vi "main.vi"(8 "error in (no error)":errorcluster) -> (0 "error out":errorcluster)   [LabVIEW 2015, in "Sample.lvlib"]
doc: "使用该模板构建用户界面事件处理设计模式。将模板应用于对话框及其它用户界面。用户也可创建并执行VI可按照与用户界面事件相同方式处理的用户定义事件。"
uses:
  Sample.lvlib
  Support/Result Panel State.ctl
  Support/UI Ref.ctl
  <vilib>/addons/database/Connection.llb/Conn ObjectReference.ctl
  Support/Configuration.ctl
  Sub VIs/Database Processing/Support/Table/Measure_Bio_Type.ctl
  Sub VIs/Database Processing/Database Processing.lvlib
  <vilib>/addons/database/NI_Database_API.lvlib
  Sub VIs/Utility VIs/Utility VIs.lvlib
  Sub VIs/Boimetry Processing/Boimetry Processing.lvlib
panel:
  in  "计算":bool caption="开始"
  in  "开始":bool
  in  "编辑":bool caption="开始"
  out "出生日期":string
  out "性别":string
  out "姓名":string
  in  "OD Summary":string[][](table)
  in  "OD parameter list":string[][](table)
  out "Image":T1(plugin-control)
  out "Ascan Display":dbl[](graph)
  in  "OS Summary":string[][](table)
  in  "OS parameter list":string[][](table)
  out "状态栏":string
  in  "stop":bool caption="停止"
  # "WJ90000生物参数测量仪"
  # "OD"
  # "OS"
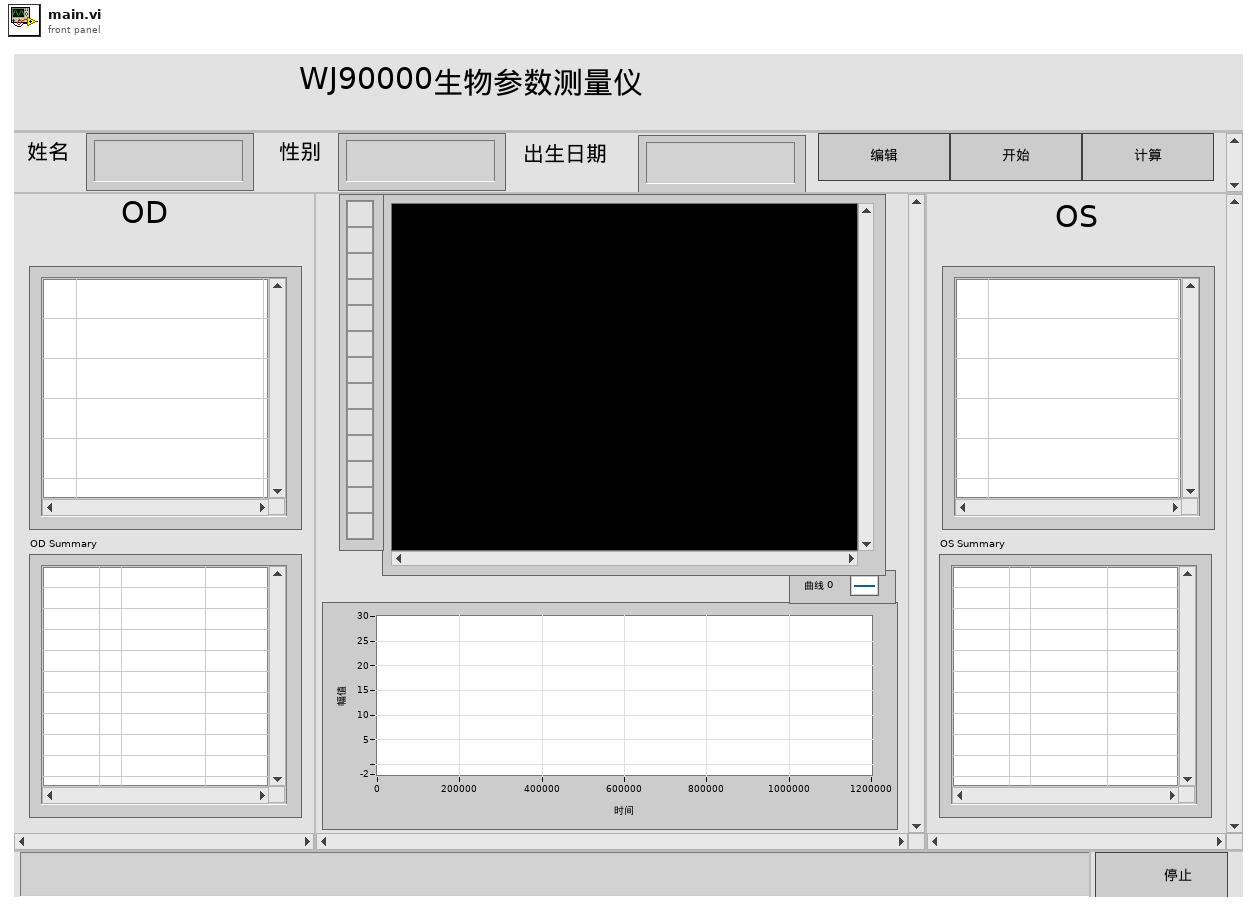
[diagram p1: front panel]
types:
  T1 = typedef "IMAQ Image.ctl" = refnum<image>
  T2 = typedef "Sample.lvlib/Configuration.ctl" = cluster{"Measure_No":i64, "Patient_ID":i64, "Oridinal":i64, "Display Parameter":enum16{"CCT", "ACD", "LT", "RT", "AL", "PD", "WTW", "K_flat", "K_steep", "K_AST"}}
  T3 = typedef "NI_Database_API.lvlib/Conn ObjectReference.ctl" = refnum<k1>
  T4 = typedef "Sample.lvlib/UI Ref.ctl" = cluster{"编辑引用句柄":refnum<vi>, "开始引用句柄":refnum<vi>, "停止引用句柄":refnum<vi>, "Ascan引用句柄":refnum<vi>, "OD Summary引用句柄":refnum<vi>, "OS Summary引用句柄":refnum<vi>, "OD parameter list引用句柄":refnum<vi>, "OS parameter list引用句柄":refnum<vi>}
  T5 = typedef "Sample.lvlib/Result Panel State.ctl" = enum16{"Initialize", "Connect Database", "Select Database", "Register", "Wait For Event", "Start", "Calculation", "Display Result", "OS Summary Update", "OS Parameter List Update", "OD Summary Update", "OD Parameter List Update", "Exit", "OD IMG Parameter List Update", "OS IMG Parameter List Update"}
  T6 = typedef "Database Processing.lvlib/Measure_Bio_Type.ctl" = cluster{"Measure_No":i64, "Measure_Time":string, "Patient_ID":i64}
  T7 = enum16{"CCT", "ACD", "LT", "RT", "AL", "PD", "WTW", "K_flat", "K_steep", "K_AST"}
  T8 = typedef "LVPoint32TypeDef.ctl" = cluster{"Horizontal":i32, "Vertical":i32}
  T9 = typedef "LVRowAndColumnTypeDef.ctl" = cluster{"Row":i32, "Column":i32}
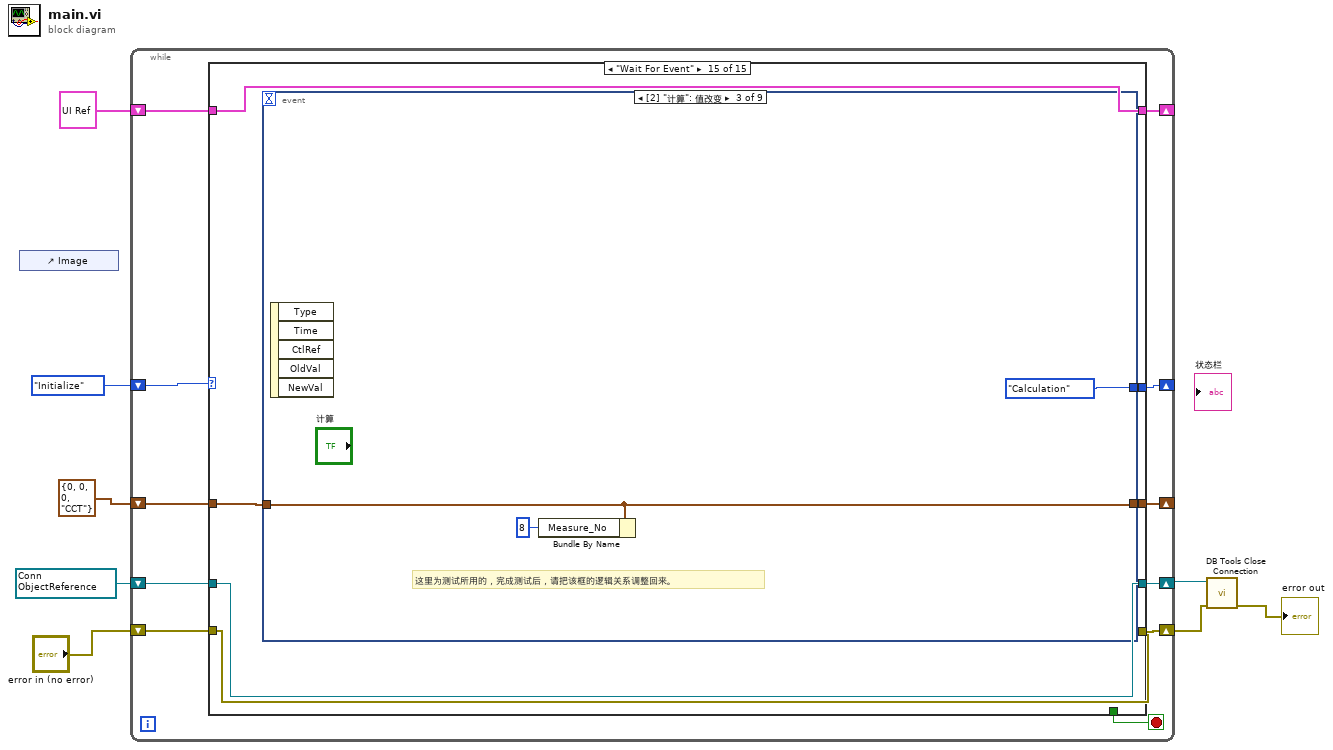
[diagram p0: block diagram]
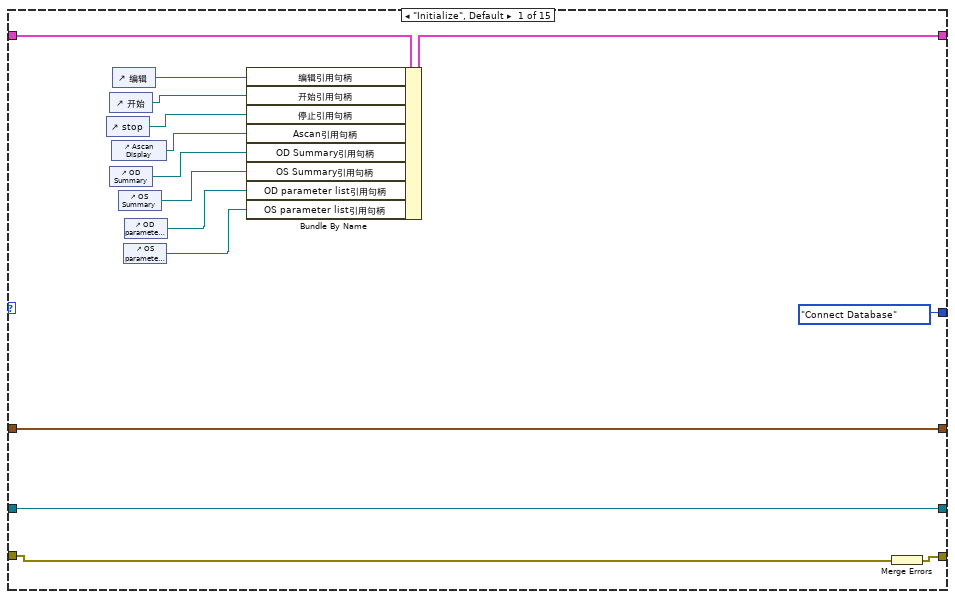
[diagram p2: hidden frame]
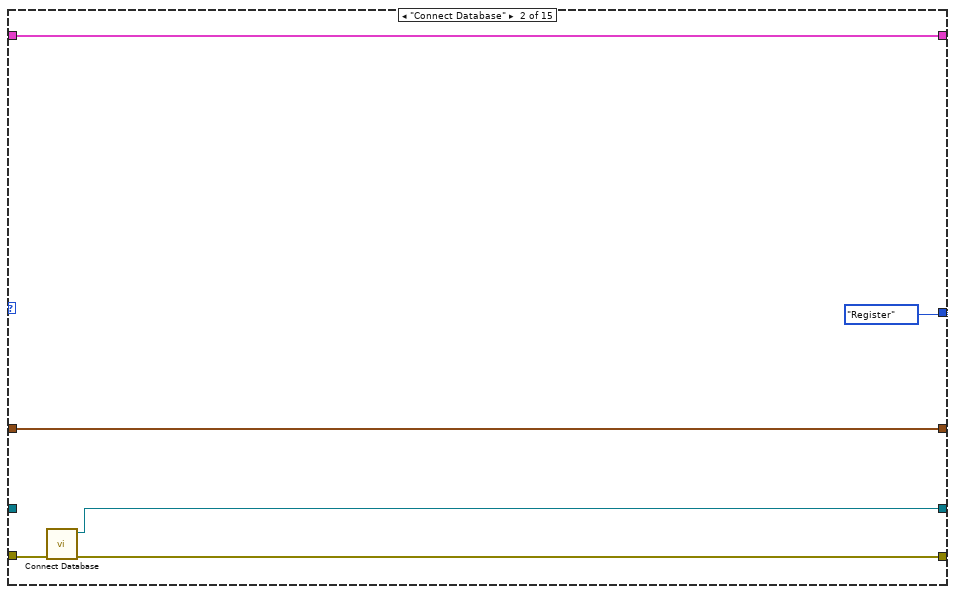
[diagram p3: hidden frame]
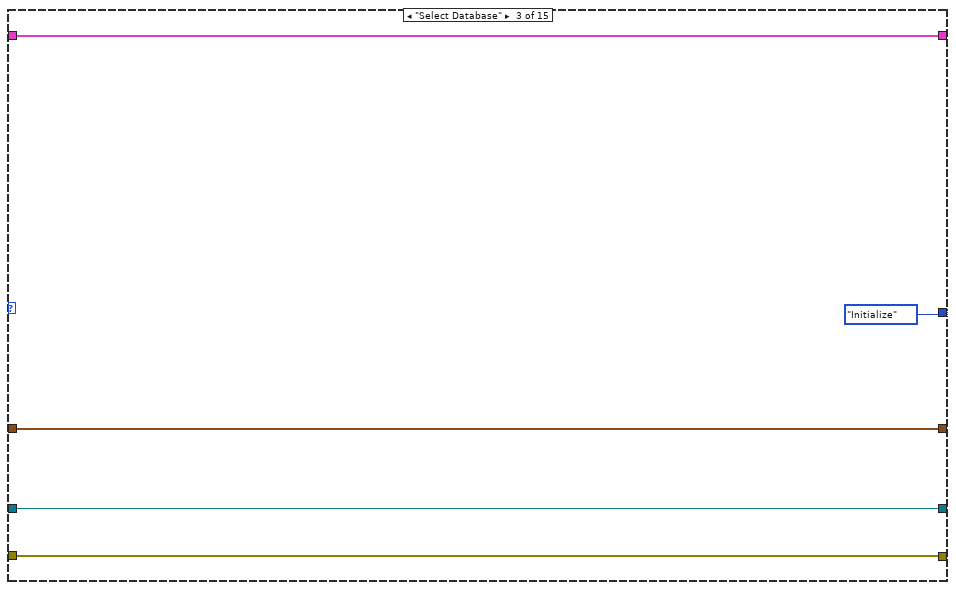
[diagram p4: hidden frame]
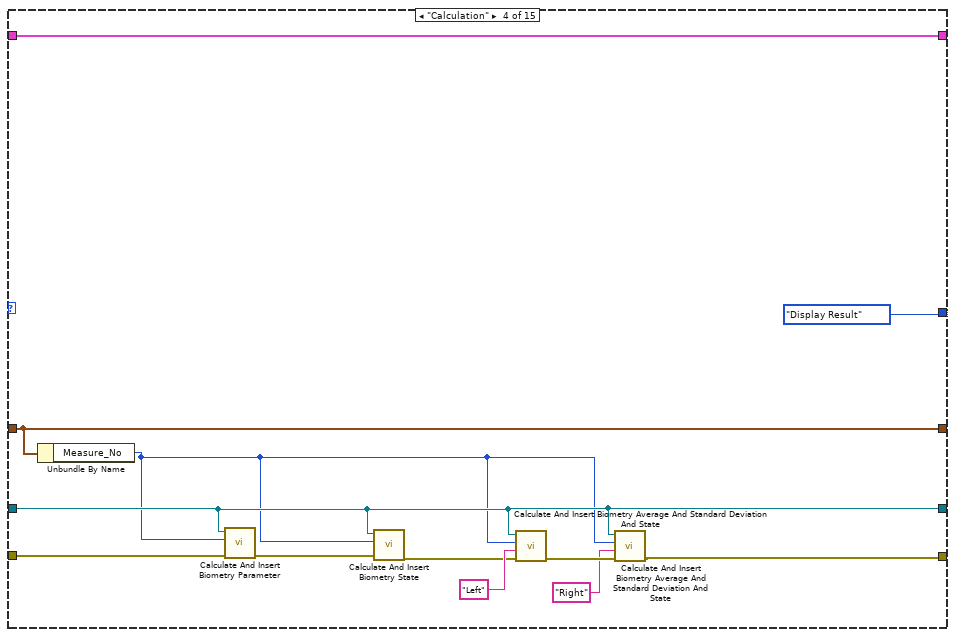
[diagram p5: hidden frame]
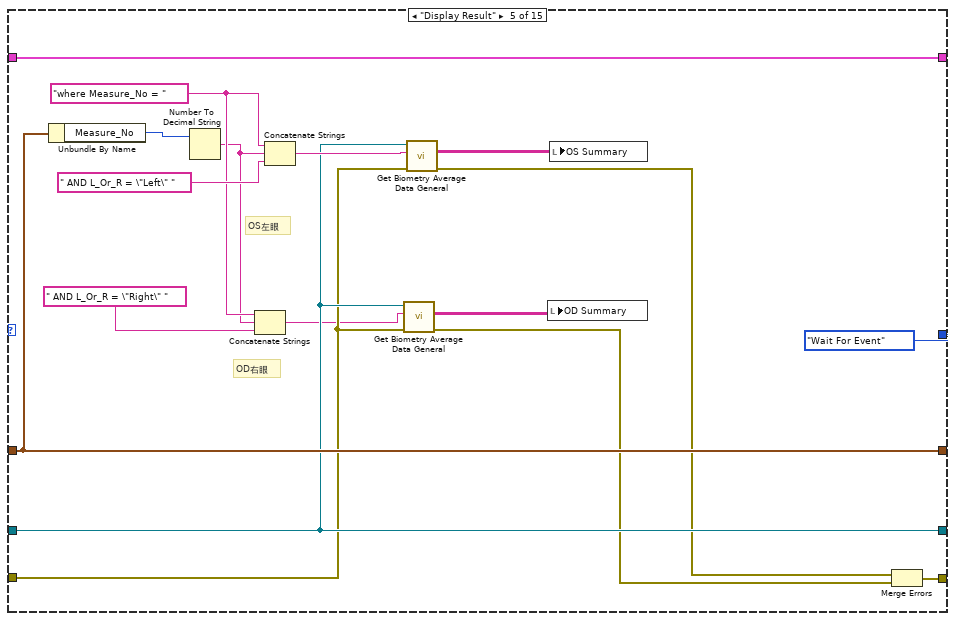
[diagram p6: hidden frame]
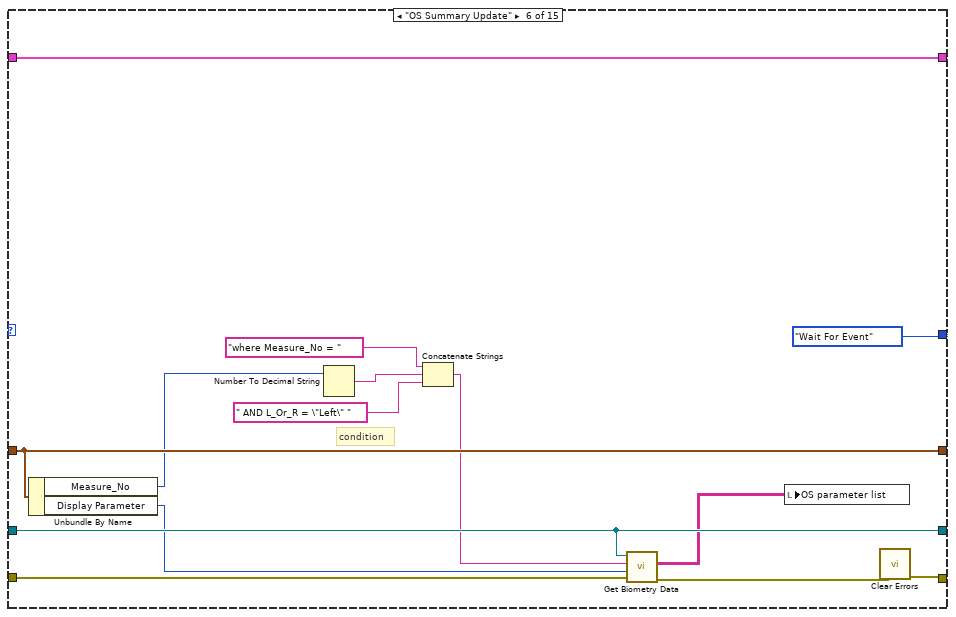
[diagram p7: hidden frame]
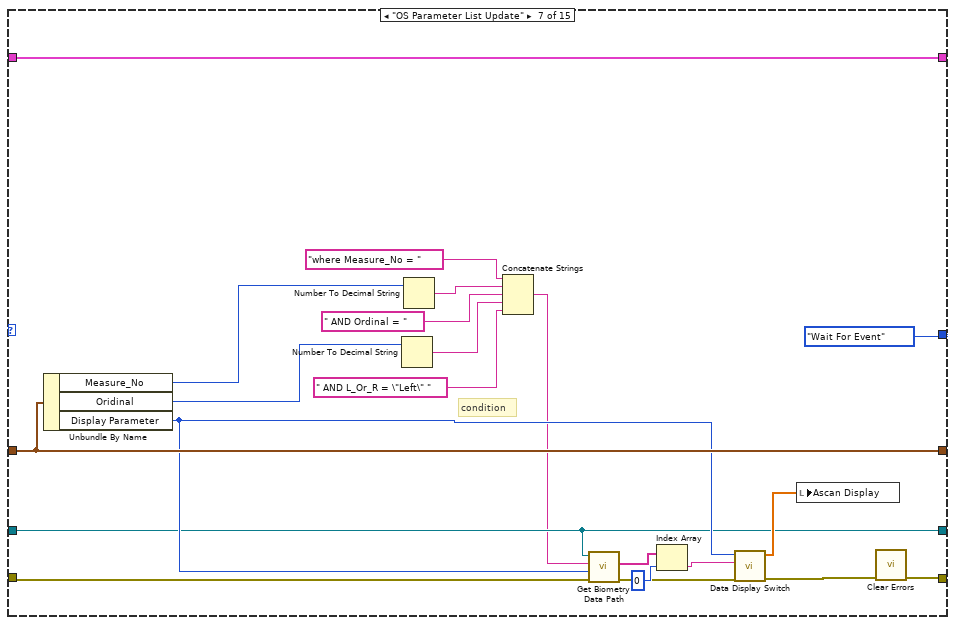
[diagram p8: hidden frame]
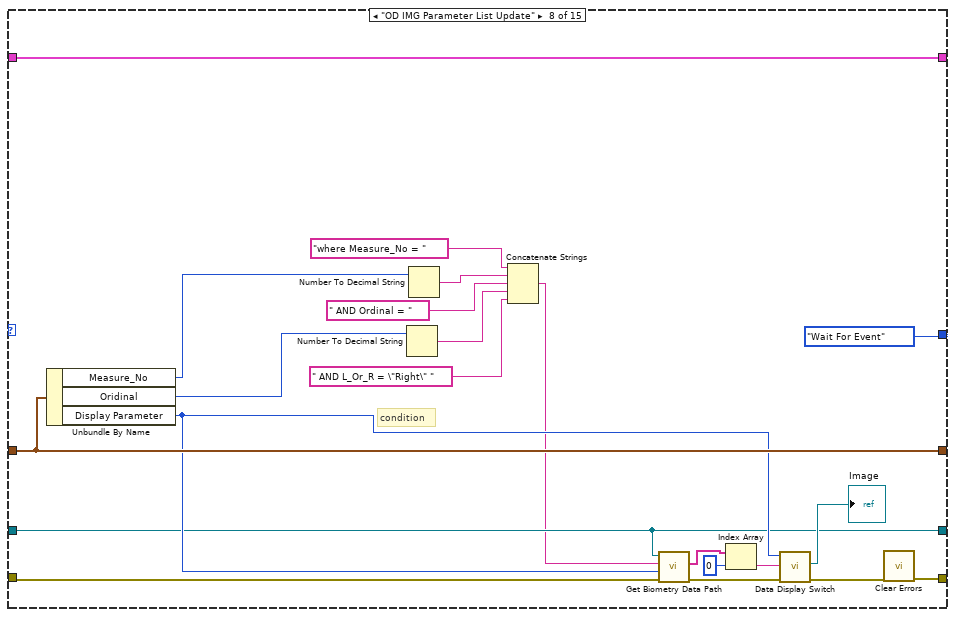
[diagram p9: hidden frame]
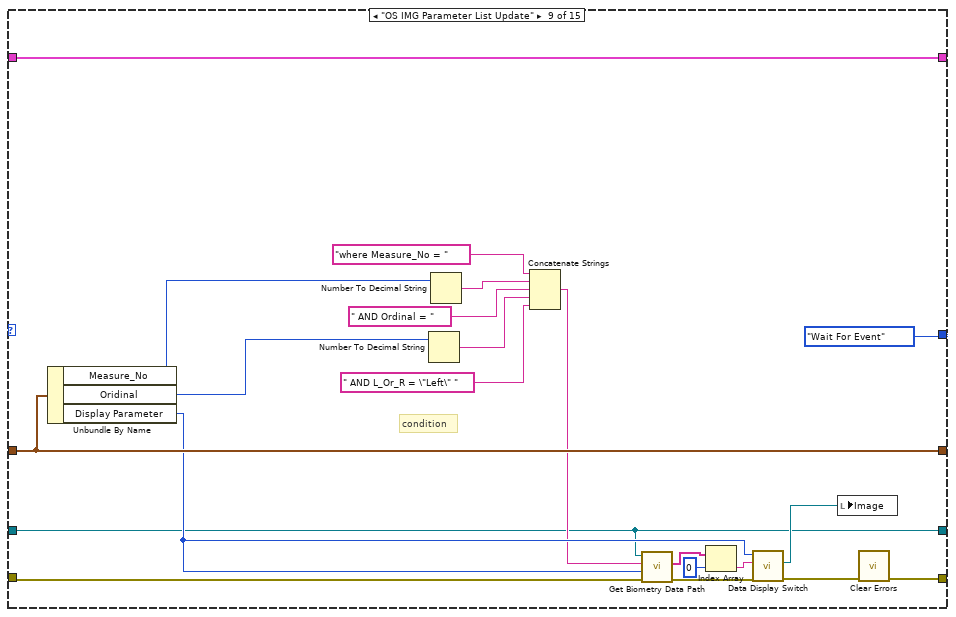
[diagram p10: hidden frame]
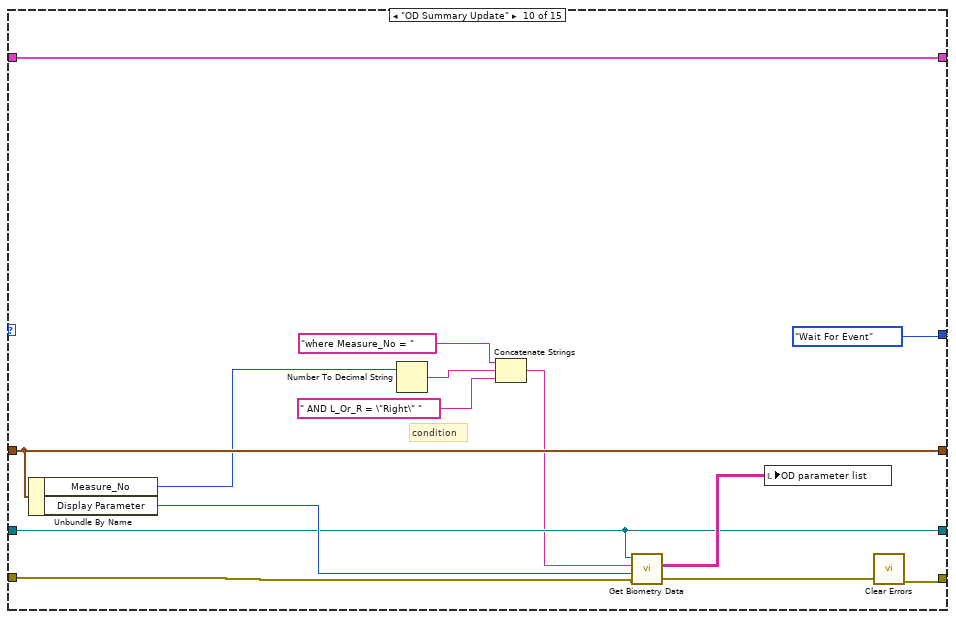
[diagram p11: hidden frame]
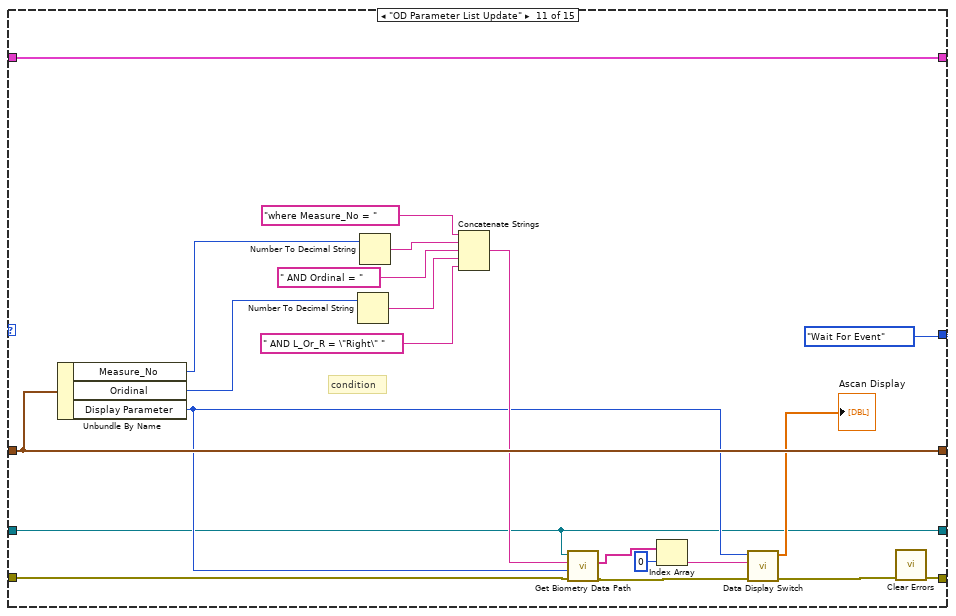
[diagram p12: hidden frame]
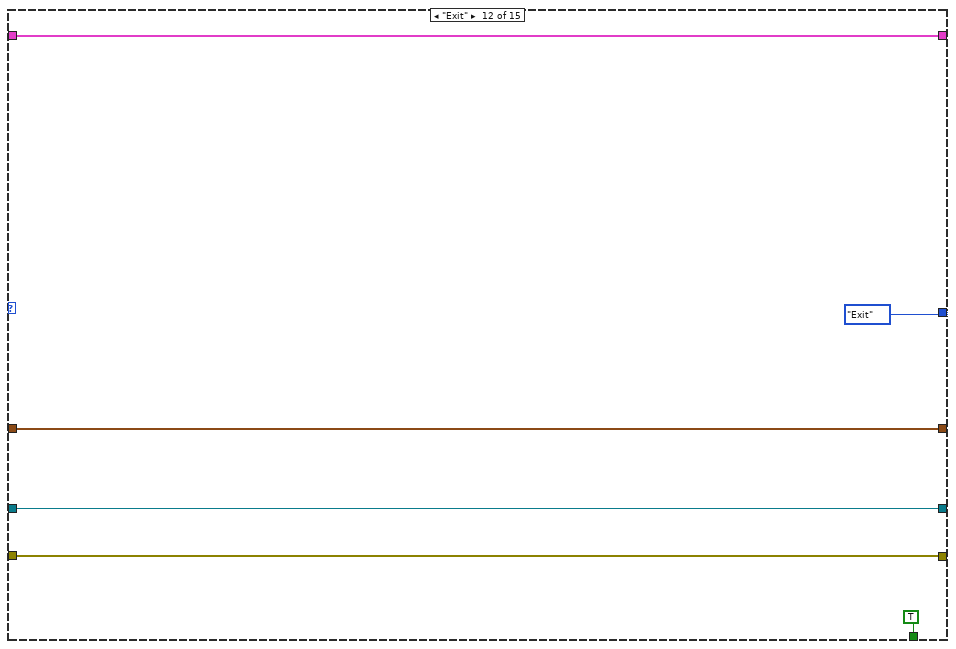
[diagram p13: hidden frame]
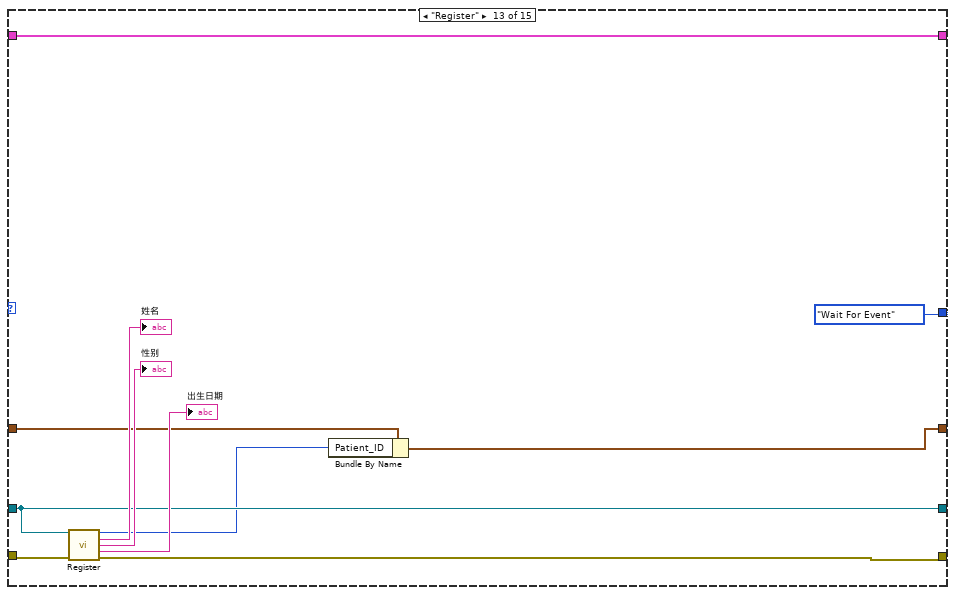
[diagram p14: hidden frame]
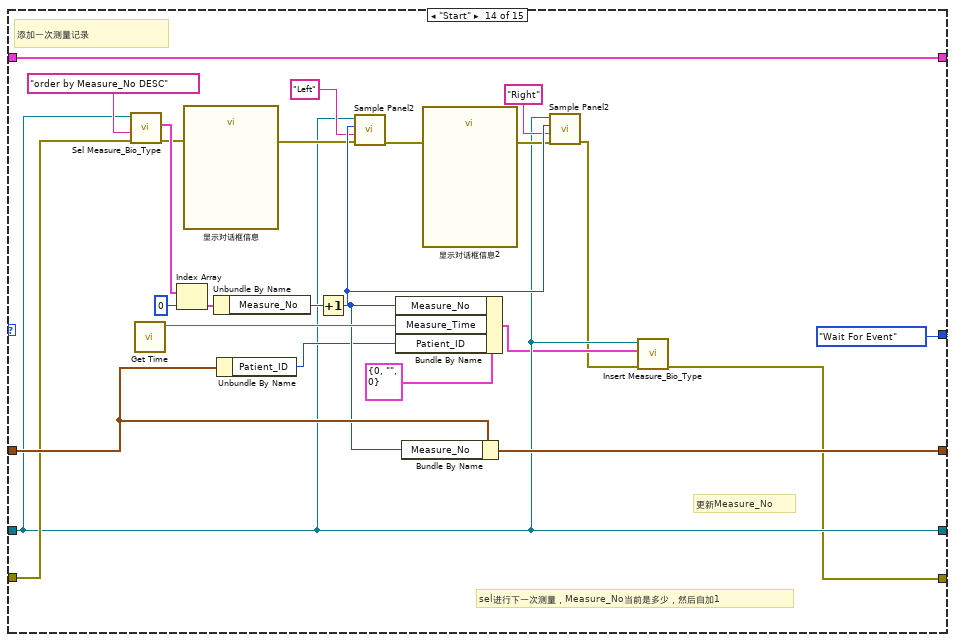
[diagram p15: hidden frame]
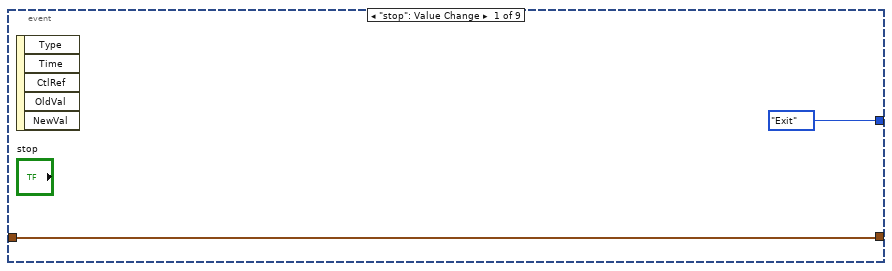
[diagram p16: hidden frame]
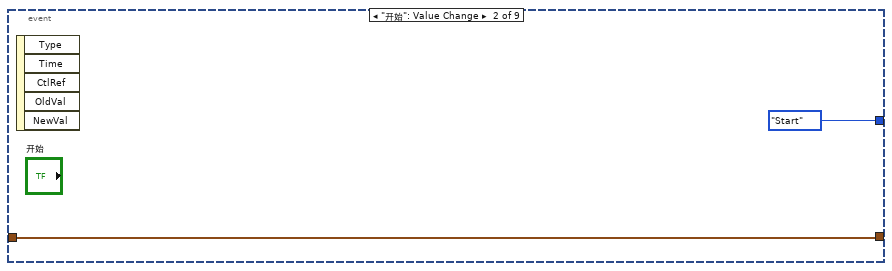
[diagram p17: hidden frame]
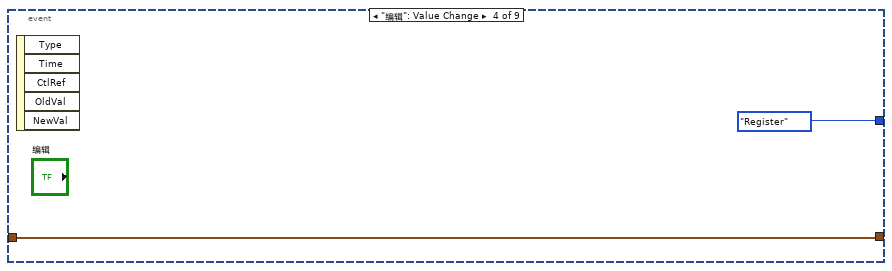
[diagram p18: hidden frame]
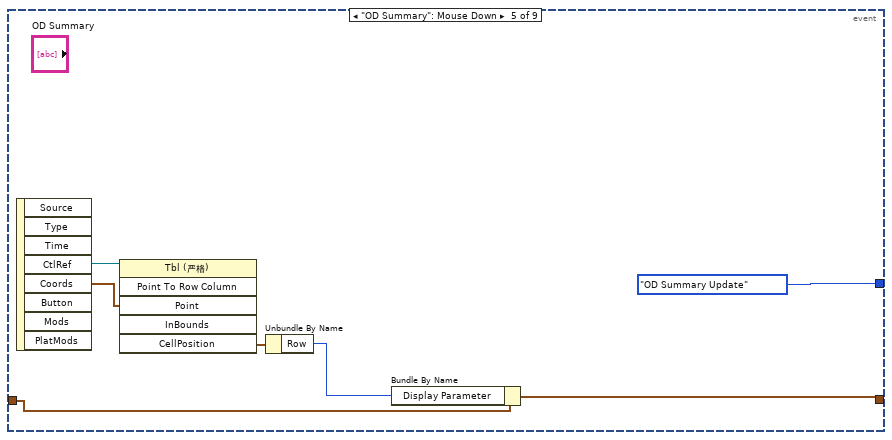
[diagram p19: hidden frame]
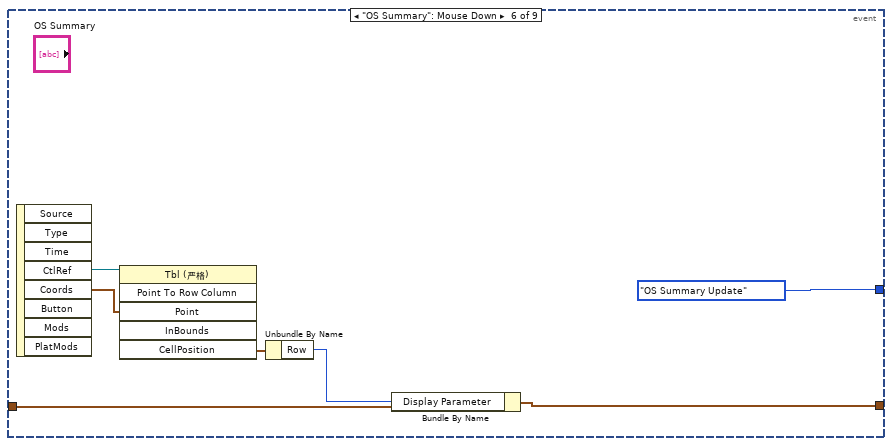
[diagram p20: hidden frame]
diagram:
  w5 = T3 refnum items=["Connection"] ("connection reference")
  n1 = control-ref of="Image"() -> ()  [unwired: 1 out]
  n2 = while {
    shift-right: [w17] -> _
    shift-left: T4 {"编辑引用句柄"=refnum, "开始引用句柄"=refnum, "停止引用句柄"=refnum, "Ascan引用句柄"=refnum, "OD Summary引用句柄"=refnum, "OS Summary引用句柄"=refnum, "OD parameter list引用句柄"=refnum, "OS parameter list引用句柄"=refnum} ("UI State") -> [w16]
    shift-right: [w15] -> _
    shift-left: Result_Panel_State."Initialize" ("State") -> [w18]
    shift-right: [w13] -> w3
    shift-left: "error in (no error)" -> [w14]
    shift-right: [w11] -> _
    shift-left: T2 {"Measure_No"=0, "Patient_ID"=0, "Oridinal"=0, "Display Parameter"=enum."CCT"} ("Configuration") -> [w12]
    shift-right: [w9] -> w4
    shift-left: w5 -> [w10]
    stop <- w19 stop-if-true
    n3 = case shown="\"Wait For Event\"" w18 {
      tunnel: [_ _ _ _ _ _ _ _ _ _ _ TRUE ("stop") _ _ _] -> w19
      tunnel: [w29 w37 w45 w57 w66 w85 w109 w130 w151 w162 w186 w192 w201 w226 w230] -> w17
      tunnel: w16 -> [w34 w37 w45 w57 w66 w85 w109 w130 w151 w162 w186 w192 w201 w226 w230]
      tunnel: [Result_Panel_State."Connect Database" ("State") Result_Panel_State."Register" ("State") Result_Panel_State."Initialize" ("State") Result_Panel_State."Display Result" ("State") Result_Panel_State."Wait For Event" ("State") Result_Panel_State."Wait For Event" ("State") Result_Panel_State."Wait For Event" ("State") Result_Panel_State."Wait For Event" ("State") Result_Panel_State."Wait For Event" ("State") Result_Panel_State."Wait For Event" ("State") Result_Panel_State."Wait For Event" ("State") Result_Panel_State."Exit" ("State") Result_Panel_State."Wait For Event" ("State") Result_Panel_State."Wait For Event" ("State") w233] -> w15
      tunnel: w14 -> [w20 w39 w41 w55 w63 w84 w101 w119 w140 w160 w172 w188 w202 w211 w232]
      tunnel: [w21 w38 w41 w49 w73 w86 w103 w124 w145 w163 w180 w188 w196 w204 w232] -> w13
      tunnel: w12 -> [w27 w35 w43 w54 w68 w87 w107 w128 w149 w164 w184 w190 w195 w224 w229]
      tunnel: [w27 w35 w43 w54 w68 w87 w107 w128 w149 w164 w184 w190 w193 w225 w228] -> w11
      tunnel: w10 -> [w26 _ w42 w48 w64 w82 w99 w118 w131 w157 w168 w189 w197 w207 w231]
      tunnel: [w26 w36 w42 w48 w64 w82 w99 w118 w131 w157 w168 w189 w197 w207 w231] -> w9
      frame "Initialize", Default {
        n4 = control-ref of="stop"() -> (w31:refnum<vi>)
        n5 = control-ref of="开始"() -> (w32:refnum<vi>)
        n6 = control-ref of="OD Summary"() -> (w25:refnum<vi>)
        n7 = control-ref of="Ascan Display"() -> (w30:refnum<vi>)
        n8 = control-ref of="编辑"() -> (w33:refnum<vi>)
        n9 = control-ref of="OS Summary"() -> (w24:refnum<vi>)
        n10 = control-ref of="OS parameter list"() -> (w22:refnum<vi>)
        n11 = control-ref of="OD parameter list"() -> (w23:refnum<vi>)
        n12 = Bundle By Name(cluster=w34, "编辑引用句柄"=w33, "开始引用句柄"=w32, "停止引用句柄"=w31, "Ascan引用句柄"=w30, "OD Summary引用句柄"=w25, "OS Summary引用句柄"=w24, "OD parameter list引用句柄"=w23, "OS parameter list引用句柄"=w22) -> (w29:T4)
        n13 = Merge Errors(w20) -> (w21:errorcluster)
      }
      frame "Connect Database" {
        n14 = call "Connect Database.vi"("error in (no error)"=w39) -> ("error out"=w38:errorcluster, "connection reference"=w36:T3)  [unwired: 9 in]
      }
      frame "Select Database" {
      }
      frame "Calculation" {
        n15 = Unbundle By Name(w54) -> ("Measure_No"=w47:i64)
        n16 = call "Calculate And Insert Biometry Parameter.vi"("error in (no error)"=w55, "Measure_No"=w47, "connection reference"=w48) -> ("error out"=w53:errorcluster)  [unwired: 8 in]
        n17 = call "Calculate And Insert Biometry State.vi"("error in (no error)"=w53, "Measure_No"=w47, "connection reference"=w48) -> ("error out"=w51:errorcluster)  [unwired: 8 in]
        n18 = call "Calculate And Insert Biometry Average And Standard Deviation And State.vi"("error in (no error)"=w51, "L_Or_R"="Left", "Measure_No"=w47, "connection reference"=w48) -> ("error out"=w50:errorcluster)  [unwired: 7 in]
        n19 = call "Calculate And Insert Biometry Average And Standard Deviation And State.vi"("error in (no error)"=w50, "L_Or_R"="Right", "Measure_No"=w47, "connection reference"=w48) -> ("error out"=w49:errorcluster)  [unwired: 7 in]
      }
      frame "Display Result" {
        w71 = "where Measure_No = " ("字符串")
        # "OD右眼"
        # "OS左眼"
        n20 = Unbundle By Name(w68) -> ("Measure_No"=w67:i64)
        n21 = Number To Decimal String(number=w67) -> (decimal integer string=w70:string)  [unwired: 1 in]
        n22 = Concatenate Strings(w71, w70, " AND L_Or_R = \"Right\" " ("字符串")) -> (w62:string)
        n23 = Concatenate Strings(w71, w70, " AND L_Or_R = \"Left\" " ("字符串")) -> (w65:string)
        n24 = call "Get Biometry Average Data General.vi"("error in (no error)"=w63, "condition"=w62, "connection reference"=w64) -> ("error out"=w58:errorcluster, "Data Output"=w60:string[][])  [unwired: 7 in]
        n25 = call "Get Biometry Average Data General.vi"("error in (no error)"=w63, "condition"=w65, "connection reference"=w64) -> ("error out"=w59:errorcluster, "Data Output"=w61:string[][])  [unwired: 7 in]
        n26 = local write "OD Summary"(w60) -> ()
        n27 = local write "OS Summary"(w61) -> ()
        n28 = Merge Errors(w59, w58) -> (w73:errorcluster)
      }
      frame "OS Summary Update" {
        # "condition"
        n29 = Unbundle By Name(w87) -> ("Measure_No"=w76:i64, "Display Parameter"=w81:T7)
        n30 = Number To Decimal String(number=w76) -> (decimal integer string=w78:string)  [unwired: 1 in]
        n31 = Concatenate Strings("where Measure_No = ", w78, " AND L_Or_R = \"Left\" " ("字符串")) -> (w75:string)
        n32 = call "Get Biometry Data.vi"("error in (no error)"=w84, "Display Parameter"=w81, "condition"=w75, "connection reference"=w82) -> ("error out"=w83:errorcluster, "Data Output"=w80:string[][])  [unwired: 6 in]
        n33 = local write "OS parameter list"(w80) -> ()
        n34 = call <vilib>:"Clear Errors.vi"("error in (no error)"=w83) -> ("error out"=w86:errorcluster)  [unwired: 5 in, 1 out]
      }
      frame "OS Parameter List Update" {
        # "condition"
        n35 = Unbundle By Name(w107) -> ("Measure_No"=w90:i64, "Oridinal"=w89:i64, "Display Parameter"=w100:T7)
        n36 = Number To Decimal String(number=w89) -> (decimal integer string=w95:string)  [unwired: 1 in]
        n37 = Number To Decimal String(number=w90) -> (decimal integer string=w97:string)  [unwired: 1 in]
        n38 = Concatenate Strings("where Measure_No = ", w97, " AND Ordinal = " ("字符串"), w95, " AND L_Or_R = \"Left\" " ("字符串")) -> (w91:string)
        n39 = call "Get Biometry Data Path.vi"("error in (no error)"=w101, "Display Parameter"=w100, "condition"=w91, "connection reference"=w99) -> ("error out"=w102:errorcluster, "Data Path Output"=w93:string[])  [unwired: 6 in]
        n40 = Index Array(array=w93, index=0 ("索引")) -> (element=w92:string)
        n41 = call "Data Display Switch.vi"("error in"=w102, "Path"=w92, "Switch"=w100) -> ("error out"=w104:errorcluster, "Ascan"=w105:dbl[])  [unwired: 6 in, 1 out]
        n42 = local write "Ascan Display"(w105) -> ()
        n43 = call <vilib>:"Clear Errors.vi"("error in (no error)"=w104) -> ("error out"=w103:errorcluster)  [unwired: 5 in, 1 out]
      }
      frame "OD IMG Parameter List Update" {
        # "condition"
        n44 = Unbundle By Name(w128) -> ("Measure_No"=w112:i64, "Oridinal"=w111:i64, "Display Parameter"=w120:T7)
        n45 = Number To Decimal String(number=w111) -> (decimal integer string=w114:string)  [unwired: 1 in]
        n46 = Number To Decimal String(number=w112) -> (decimal integer string=w116:string)  [unwired: 1 in]
        n47 = Concatenate Strings("where Measure_No = ", w116, " AND Ordinal = " ("字符串"), w114, " AND L_Or_R = \"Right\" " ("字符串")) -> (w110:string)
        n48 = call "Get Biometry Data Path.vi"("error in (no error)"=w119, "Display Parameter"=w120, "condition"=w110, "connection reference"=w118) -> ("error out"=w123:errorcluster, "Data Path Output"=w122:string[])  [unwired: 6 in]
        n49 = Index Array(array=w122, index=0 ("索引")) -> (element=w121:string)
        n50 = call "Data Display Switch.vi"("error in"=w123, "Path"=w121, "Switch"=w120) -> ("error out"=w125:errorcluster, "Image Out"=→"Image":T1)  [unwired: 6 in, 1 out]
        n51 = call <vilib>:"Clear Errors.vi"("error in (no error)"=w125) -> ("error out"=w124:errorcluster)  [unwired: 5 in, 1 out]
      }
      frame "OS IMG Parameter List Update" {
        # "condition"
        n52 = Unbundle By Name(w149) -> ("Measure_No"=w133:i64, "Oridinal"=w132:i64, "Display Parameter"=w141:T7)
        n53 = Number To Decimal String(number=w132) -> (decimal integer string=w136:string)  [unwired: 1 in]
        n54 = Number To Decimal String(number=w133) -> (decimal integer string=w138:string)  [unwired: 1 in]
        n55 = Concatenate Strings("where Measure_No = ", w138, " AND Ordinal = " ("字符串"), w136, " AND L_Or_R = \"Left\" " ("字符串")) -> (w134:string)
        n56 = call "Get Biometry Data Path.vi"("error in (no error)"=w140, "Display Parameter"=w141, "condition"=w134, "connection reference"=w131) -> ("error out"=w144:errorcluster, "Data Path Output"=w143:string[])  [unwired: 6 in]
        n57 = Index Array(array=w143, index=0 ("索引")) -> (element=w142:string)
        n58 = call "Data Display Switch.vi"("error in"=w144, "Path"=w142, "Switch"=w141) -> ("error out"=w146:errorcluster, "Image Out"=w147:T1)  [unwired: 6 in, 1 out]
        n59 = local write "Image"(w147) -> ()
        n60 = call <vilib>:"Clear Errors.vi"("error in (no error)"=w146) -> ("error out"=w145:errorcluster)  [unwired: 5 in, 1 out]
      }
      frame "OD Summary Update" {
        # "condition"
        n61 = Unbundle By Name(w164) -> ("Measure_No"=w152:i64, "Display Parameter"=w158:T7)
        n62 = Number To Decimal String(number=w152) -> (decimal integer string=w155:string)  [unwired: 1 in]
        n63 = Concatenate Strings("where Measure_No = ", w155, " AND L_Or_R = \"Right\" " ("字符串")) -> (w153:string)
        n64 = call "Get Biometry Data.vi"("error in (no error)"=w160, "Display Parameter"=w158, "condition"=w153, "connection reference"=w157) -> ("error out"=w161:errorcluster, "Data Output"=w159:string[][])  [unwired: 6 in]
        n65 = local write "OD parameter list"(w159) -> ()
        n66 = call <vilib>:"Clear Errors.vi"("error in (no error)"=w161) -> ("error out"=w163:errorcluster)  [unwired: 5 in, 1 out]
      }
      frame "OD Parameter List Update" {
        # "condition"
        n67 = Unbundle By Name(w184) -> ("Measure_No"=w177:i64, "Oridinal"=w175:i64, "Display Parameter"=w169:T7)
        n68 = Number To Decimal String(number=w175) -> (decimal integer string=w174:string)  [unwired: 1 in]
        n69 = Number To Decimal String(number=w177) -> (decimal integer string=w178:string)  [unwired: 1 in]
        n70 = Concatenate Strings("where Measure_No = ", w178, " AND Ordinal = " ("字符串"), w174, " AND L_Or_R = \"Right\" " ("字符串")) -> (w170:string)
        n71 = call "Get Biometry Data Path.vi"("error in (no error)"=w172, "Display Parameter"=w169, "condition"=w170, "connection reference"=w168) -> ("error out"=w171:errorcluster, "Data Path Output"=w167:string[])  [unwired: 6 in]
        n72 = Index Array(array=w167, index=0 ("索引")) -> (element=w166:string)
        n73 = call "Data Display Switch.vi"("error in"=w171, "Path"=w166, "Switch"=w169) -> ("error out"=w181:errorcluster, "Ascan"=→"Ascan Display":dbl[])  [unwired: 6 in, 1 out]
        n74 = call <vilib>:"Clear Errors.vi"("error in (no error)"=w181) -> ("error out"=w180:errorcluster)  [unwired: 5 in, 1 out]
      }
      frame "Exit" {
      }
      frame "Register" {
        n75 = call "Register.vi"("connection reference"=w197, "error in (no error)"=w202) -> ("Patient_ID"=w194:i64, "选中个人姓名"=→"姓名":string, "选中个人性别"=→"性别":string, "选中个人出生日期"=→"出生日期":string, "error out"=w196:errorcluster)  [unwired: 9 in]
        n76 = Bundle By Name(cluster=w195, "Patient_ID"=w194) -> (w193:T2)
      }
      frame "Start" {
        # "更新Measure_No"
        # "sel进行下一次测量，Measure_No当前是多少，然后自加1"
        # "添加一次测量记录"
        n77 = call "Sel Measure_Bio_Type.vi"("error in (no error)"=w211, "condition"="order by Measure_No DESC" ("Condition"), "connection reference"=w207) -> ("error out"=w208:errorcluster, "Measure_Bio_Typea"=w209:T6[])  [unwired: 7 in]
        n78 = call "Get Time.vi"() -> ("Time"=w222:string)  [unwired: 11 in]
        n79 = Index Array(array=w209, index=0 ("索引")) -> (element=w220:T6)
        n80 = call "显示对话框信息"("error in (no error)"=w208) -> ("error out"=w216:errorcluster)  [unwired: 9 in, 1 out]
        n81 = Unbundle By Name(w220) -> ("Measure_No"=w212:i64)
        n82 = Unbundle By Name(w224) -> ("Patient_ID"=w217:i64)
        n83 = Increment(x=w212) -> (x+1=w219:i64)
        n84 = call "Sample Panel2.vi"("error in (no error)"=w216, "Left Or Right"="Left" ("L_Or_R"), "Measure_No"=w219, "connection reference"=w207) -> ("error out"=w215:errorcluster)  [unwired: 7 in]
        n85 = Bundle By Name(cluster=T6 {"Measure_No"=0, "Measure_Time"="", "Patient_ID"=0} ("Measure_Bio_Type"), "Measure_No"=w219, "Measure_Time"=w222, "Patient_ID"=w217) -> (w206:T6)
        n86 = Bundle By Name(cluster=w224, "Measure_No"=w219) -> (w225:T2)
        n87 = call "显示对话框信息2"("error in (no error)"=w215) -> ("error out"=w214:errorcluster)  [unwired: 9 in, 1 out]
        n88 = call "Sample Panel2.vi"("error in (no error)"=w214, "Left Or Right"="Right" ("L_Or_R"), "Measure_No"=w219, "connection reference"=w207) -> ("error out"=w205:errorcluster)  [unwired: 7 in]
        n89 = call "Insert Measure_Bio_Type.vi"("error in (no error)"=w205, "Measure_Bio_Type"=w206, "connection reference"=w207) -> ("error out"=w204:errorcluster)  [unwired: 8 in]
      }
      frame "Wait For Event" {
        n90 = event shown="[2] \"计算\": 值改变" {
          selector: _ -> [_ _ _ _ _ _ _ _ _]
          dyn-events: _ -> [_ _ _ _ _ _ _ _ _]
          timeout: _ -> [_ _ _ _ _ _ _ _ _]
          tunnel: [Result_Panel_State."Exit" ("State") Result_Panel_State."Start" ("State") Result_Panel_State."Calculation" ("State") Result_Panel_State."Register" ("State") Result_Panel_State."OD Summary Update" ("State") Result_Panel_State."OS Summary Update" ("State") w261 w271 Result_Panel_State."Exit" ("State")] -> w233
          tunnel: w229 -> [w234 w236 w238 w241 w244 w251 w260 w270 w278]
          tunnel: [w234 w236 w238 w241 w245 w252 w258 w268 w278] -> w228
          event "stop": Value Change {
            n91 = event-data() -> ()  [unwired: 1 in, 5 out]
          }
          event "开始": Value Change {
            n92 = event-data() -> ()  [unwired: 1 in, 5 out]
          }
          event "计算": Value Change {
            # "这里为测试所用的，完成测试后，请把该框的逻辑关系调整回来。"
            n93 = event-data() -> ()  [unwired: 1 in, 5 out]
            n94 = Bundle By Name(cluster=w238, "Measure_No"=i64 8) -> ()  [unwired: 1 out]
          }
          event "编辑": Value Change {
            n95 = event-data() -> ()  [unwired: 1 in, 5 out]
          }
          event "OD Summary": Mouse Down {
            n96 = event-data() -> ("CtlRef"=w248:refnum<vi>, "Coords"=w247:T8)  [unwired: 1 in, 6 out]
            n97 = invoke class="Tbl (严格)" method="Point To Row Column"(reference=w248, "Point"=w247) -> ("CellPosition"=w246:T9)  [unwired: 4 in, 5 out]
            n98 = Unbundle By Name(w246) -> ("Row"=w243:i32)
            n99 = Bundle By Name(cluster=w244, "Display Parameter"=w243) -> (w245:T2)
          }
          event "OS Summary": Mouse Down {
            n100 = event-data() -> ("CtlRef"=w255:refnum<vi>, "Coords"=w254:T8)  [unwired: 1 in, 6 out]
            n101 = invoke class="Tbl (严格)" method="Point To Row Column"(reference=w255, "Point"=w254) -> ("CellPosition"=w253:T9)  [unwired: 4 in, 5 out]
            n102 = Unbundle By Name(w253) -> ("Row"=w250:i32)
            n103 = Bundle By Name(cluster=w251, "Display Parameter"=w250) -> (w252:T2)
          }
          event "OD parameter list": Mouse Down {
            n104 = event-data() -> ("CtlRef"=w266:refnum<vi>, "Coords"=w265:T8)  [unwired: 1 in, 3 out]
            n105 = invoke class="Tbl (严格)" method="Point To Row Column"(reference=w266, "Point"=w265) -> ("CellPosition"=w264:T9)  [unwired: 4 in, 5 out]
            n106 = Unbundle By Name(w264) -> ("Row"=w263:i32)
            n107 = Increment(x=w263) -> (x+1=w259:i32)
            n108 = Bundle By Name(cluster=w260, "Oridinal"=w259) -> (w258:T2)
            n109 = Unbundle By Name(w258) -> ("Display Parameter"=w262:T7)
            n110 = call "Display Parameter Switch.vi"("L_Or_R"="OD", "Switch"=w262) -> ("State"=w261:T5)  [unwired: 7 in, 2 out]
          }
          event "OS parameter list": Mouse Down {
            n111 = event-data() -> ("CtlRef"=w276:refnum<vi>, "Coords"=w275:T8)  [unwired: 1 in, 3 out]
            n112 = invoke class="Tbl (严格)" method="Point To Row Column"(reference=w276, "Point"=w275) -> ("CellPosition"=w274:T9)  [unwired: 4 in, 5 out]
            n113 = Unbundle By Name(w274) -> ("Row"=w272:i32)
            n114 = Increment(x=w272) -> (x+1=w269:i32)
            n115 = Bundle By Name(cluster=w270, "Oridinal"=w269) -> (w268:T2)
            n116 = Unbundle By Name(w268) -> ("Display Parameter"=w273:T7)
            n117 = call "Display Parameter Switch.vi"("L_Or_R"="OS", "Switch"=w273) -> ("State"=w271:T5)  [unwired: 7 in, 2 out]
          }
          event Timeout {
            n118 = event-data() -> ()  [unwired: 1 in, 3 out]
          }
        }
      }
    }
  }
  n119 = call <vilib>:"DB Tools Close Connection.vi"("error in (no error)"=w3, "connection reference"=w4) -> ("error out"=→"error out":errorcluster)  [unwired: 5 in]
